vi "rqcBob Read PD Detection FIFO.vi"   [LabVIEW 2018]
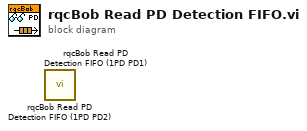
[diagram p0: block diagram]
diagram:
  n1 = call "rqcBob Read PD Detection FIFO (1PD PD2).vi"() -> ()  [unwired: 8 in, 4 out]
  n2 = call "rqcBob Read PD Detection FIFO (1PD PD1).vi"() -> ()  [unwired: 8 in, 4 out]
